vi "Dummy ARGB Data.vi"(8 "error in (no error)":errorcluster) -> (0 "error out":errorcluster, 2 "Data Value Reference out":refnum<data-value>, 3 "Data":u32[][](array[numeric]) format="%x")   [LabVIEW 2020, in "g_ar_toolkit.test.lvlib" / "Image.lvclass"]
uses:
  Image.lvclass
  g_ar_toolkit.image/CreateEmptyImageARGB.vi
  g_ar_toolkit.image/CopyArrayToImageARGB.vi
  g_ar_toolkit.image/CreateEmptyImageARGB.vi/3321fa97-f432-4e1e-8db9-a0df79aed21b.vi
  g_ar_toolkit.image/CopyArrayToImageARGB.vi/26c70cee-9332-41f4-9755-08948a885cbe.vi
  g_ar_toolkit.image/ARGBColourToU32.vi
  <vilib>/Utility/error.llb/Error Cluster From Error Code.vi
  Image.lvclass/Image.ctl
  g_ar_toolkit.image/g_ar_toolkit.image.lvlib
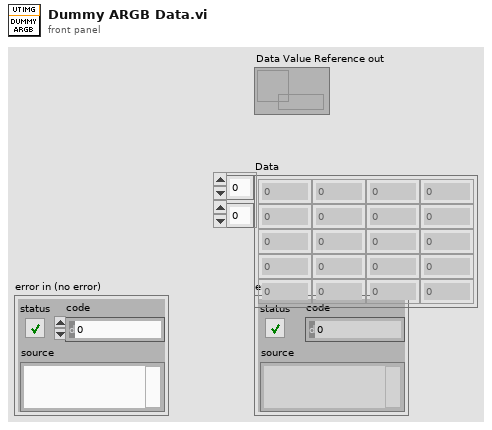
[diagram p1: front panel]
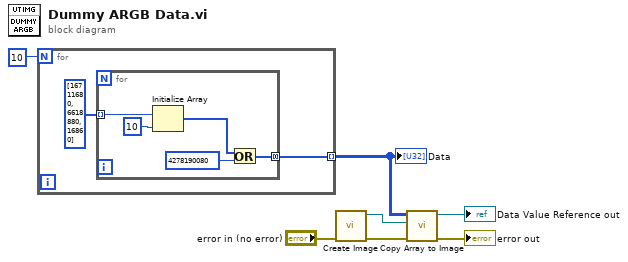
[diagram p0: block diagram]
diagram:
  n1 = for {
    N: 10 -> [_]
    tunnel: [w8] -> w4 mode=indexing
    n2 = for {
      tunnel: u32[] [16711680, 6618880, 16860] -> [w14] mode=indexing
      tunnel: [w11] -> w8 mode=concatenating
      n3 = Initialize Array(w14, 10 ("dimension size")) -> (w12:u32[])
      n4 = Or(x=w12, y=u32 4278190080) -> (x .or. y?=w11:u32[])
    }
  }
  "Data" <- w4
  n5 = call-poly "Create Image.vi"("error in (no error)"="error in (no error)") -> ("error out"=w6:errorcluster, "New ARGB Image"=w1:refnum<data-value>)  [unwired: 9 in]
  n6 = call-poly "Copy Array to Image.vi"("error in (no error)"=w6, "ARGB Image Destination"=w1, "Source"=w4) -> ("error out"=→"error out":errorcluster, "ARGB Image Destination (Duplicate)"=→"Data Value Reference out":refnum<data-value>)  [unwired: 7 in]
